vi "Day 6 Puzzle 2.vi"(11 "Path":path) -> ()   [LabVIEW 2021]
uses:
  <vilib>/Utility/file.llb/Read Delimited Spreadsheet (string).vi
panel:
  out "Array 4":bool[](array[boolean])
  out "Array 3":bool[](array[boolean])
  out "Array 2":string[](array[string])
  out "String":string
  out "Array":string[](array[string])
  out "Numeric":i32
  out "element":string
  out "all rows":string[][](array[string])
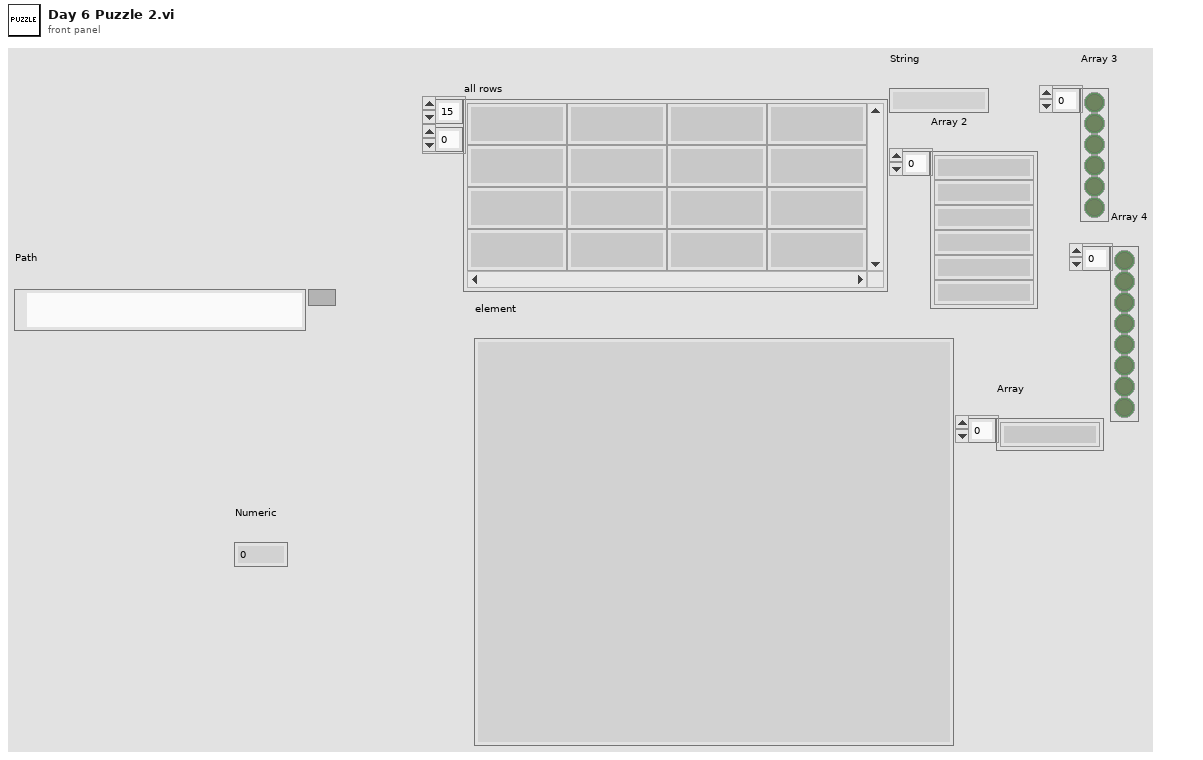
[diagram p1: front panel]
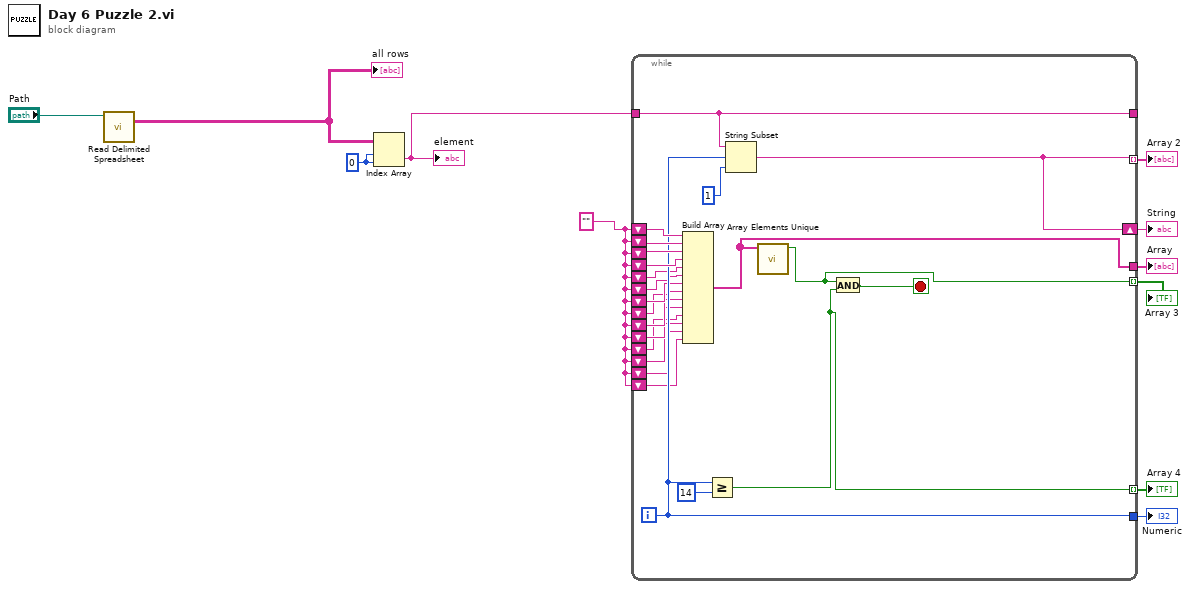
[diagram p0: block diagram]
diagram:
  w1 = "" ("String")
  w9 = 0 ("disabled index (col)")
  n1 = call-poly <vilib>:"Read Delimited Spreadsheet.vi"("file path (dialog if empty)"="Path") -> ("all rows"=w10:string[][])  [unwired: 9 in, 5 out]
  "all rows" <- w10
  n2 = Index Array(array=w10, index (row)=w9, index (col)=w9) -> (element=w8:string)
  "element" <- w8
  n3 = while {
    shift-right: [w24] -> w5
    shift-left: w1 -> [w33]
    shift-left: w1 -> [w30]
    shift-left: w1 -> [w31]
    shift-left: w1 -> [w32]
    tunnel: [w26] -> w7
    tunnel: [w27] -> w6
    tunnel: w8 -> [w29]
    tunnel: [w29] -> _
    tunnel: [w24] -> w4 mode=indexing
    tunnel: [w23] -> w3 mode=indexing
    tunnel: [w22] -> w2 mode=indexing
    shift-left: w1 -> [w21]
    shift-left: w1 -> [w20]
    shift-left: w1 -> [w19]
    shift-left: w1 -> [w18]
    shift-left: w1 -> [w17]
    shift-left: w1 -> [w16]
    shift-left: w1 -> [w15]
    shift-left: w1 -> [w14]
    shift-left: w1 -> [w13]
    shift-left: w1 -> [w12]
    i -> [w26]
    stop <- w25 stop-if-true
    n4 = Build Array(w33, w32, w31, w30, w21, w20, w19, w18, w17, w16, w15, w14, w13, w12) -> (w27:string[])
    n5 = Greater Or Equal?(x=w26, y=14) -> (x >= y?=w22:bool)
    n6 = String Subset(string=w29, offset (0)=w26, length (rest)=1 ("length (rest)")) -> (substring=w24:string)
    n7 = call "Array Elements Unique"("Array"=w27) -> ("result"=w23:bool)  [unwired: 10 in]
    n8 = And(x=w23, y=w22) -> (x .and. y?=w25:bool)
  }
  "Numeric" <- w7
  "Array" <- w6
  "String" <- w5
  "Array 2" <- w4
  "Array 3" <- w3
  "Array 4" <- w2
